vi "VI Tree.vi"   [LabVIEW 2010, in "Lake Shore 335.lvlib"]
doc: "This is the instrument driver for the Lake Shore Model 335 Temperature Controller. The VI Tree displays all the user-callable VIs of the instrument driver in an organized table."
uses:
  <instrlib>/Lake Shore 335/Lake Shore 335.lvlib
  <instrlib>/Lake Shore 335/Public/Data/Sensor Data (Single Reading).vi
panel:
  # "(c) 2011 Lake Shore Cryotronics Inc.  ALL RIGHTS RESERVED."
  # "SEE DIAGRAM\nFOR VI TREE."
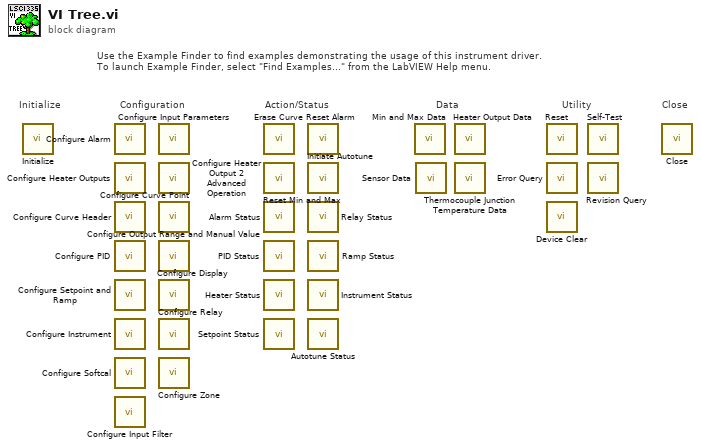
[diagram p0: block diagram]
diagram:
  # "Configuration"
  # "Utility"
  # "Data"
  # "Action/Status"
  # "Close"
  # "Initialize"
  # "Use the Example Finder to find examples demonstrating the usage of this instrument driver.\nTo launch Example Finder, select \"Find Examples...\" from the LabVIEW Help menu."
  n1 = call <instrlib>:"Initialize.vi"() -> ()  [unwired: 10 in, 2 out]
  n2 = call <instrlib>:"Configure Alarm.vi"() -> ()  [unwired: 14 in, 2 out]
  n3 = call <instrlib>:"Configure Heater Outputs.vi"() -> ()  [unwired: 18 in, 2 out]
  n4 = call <instrlib>:"Configure Curve Header.vi"() -> ()  [unwired: 14 in, 2 out]
  n5 = call <instrlib>:"Configure PID.vi"() -> ()  [unwired: 14 in, 2 out]
  n6 = call <instrlib>:"Configure Setpoint and Ramp.vi"() -> ()  [unwired: 14 in, 2 out]
  n7 = call <instrlib>:"Configure Instrument.vi"() -> ()  [unwired: 14 in, 2 out]
  n8 = call <instrlib>:"Configure Softcal.vi"() -> ()  [unwired: 14 in, 2 out]
  n9 = call <instrlib>:"Configure Input Filter.vi"() -> ()  [unwired: 14 in, 2 out]
  n10 = call <instrlib>:"Configure Input Parameters.vi"() -> ()  [unwired: 14 in, 2 out]
  n11 = call <instrlib>:"Configure Heater Output 2 Advanced Operation.vi"() -> ()  [unwired: 14 in, 2 out]
  n12 = call <instrlib>:"Configure Curve Point.vi"() -> ()  [unwired: 14 in, 2 out]
  n13 = call <instrlib>:"Configure Output Range and Manual Value.vi"() -> ()  [unwired: 14 in, 2 out]
  n14 = call <instrlib>:"Configure Display.vi"() -> ()  [unwired: 14 in, 2 out]
  n15 = call <instrlib>:"Configure Relay.vi"() -> ()  [unwired: 14 in, 2 out]
  n16 = call <instrlib>:"Configure Zone.vi"() -> ()  [unwired: 18 in, 2 out]
  n17 = call <instrlib>:"Erase Curve.vi"() -> ()  [unwired: 10 in, 2 out]
  n18 = call <instrlib>:"Reset Min and Max.vi"() -> ()  [unwired: 10 in, 2 out]
  n19 = call <instrlib>:"Alarm Status.vi"() -> ()  [unwired: 8 in, 4 out]
  n20 = call <instrlib>:"PID Status.vi"() -> ()  [unwired: 7 in, 5 out]
  n21 = call <instrlib>:"Heater Status.vi"() -> ()  [unwired: 7 in, 5 out]
  n22 = call <instrlib>:"Setpoint Status.vi"() -> ()  [unwired: 9 in, 3 out]
  n23 = call <instrlib>:"Reset Alarm.vi"() -> ()  [unwired: 10 in, 2 out]
  n24 = call <instrlib>:"Initiate Autotune.vi"() -> ()  [unwired: 14 in, 2 out]
  n25 = call <instrlib>:"Relay Status.vi"() -> ()  [unwired: 9 in, 3 out]
  n26 = call <instrlib>:"Ramp Status.vi"() -> ()  [unwired: 7 in, 5 out]
  n27 = call <instrlib>:"Instrument Status.vi"() -> ()  [unwired: 5 in, 7 out]
  n28 = call <instrlib>:"Autotune Status.vi"() -> ()  [unwired: 6 in, 6 out]
  n29 = call <instrlib>:"Min and Max Data.vi"() -> ()  [unwired: 8 in, 4 out]
  n30 = call-poly <instrlib>:"Sensor Data.vi"() -> ()  [unwired: 9 in, 3 out]
  n31 = call <instrlib>:"Heater Output Data.vi"() -> ()  [unwired: 9 in, 3 out]
  n32 = call <instrlib>:"Thermocouple Junction Temperature Data.vi"() -> ()  [unwired: 9 in, 3 out]
  n33 = call <instrlib>:"Reset.vi"() -> ()  [unwired: 10 in, 2 out]
  n34 = call <instrlib>:"Error Query.vi"() -> ()  [unwired: 9 in, 3 out]
  n35 = call <instrlib>:"Device Clear.vi"() -> ()  [unwired: 10 in, 2 out]
  n36 = call <instrlib>:"Self-Test.vi"() -> ()  [unwired: 8 in, 4 out]
  n37 = call <instrlib>:"Revision Query.vi"() -> ()  [unwired: 5 in, 7 out]
  n38 = call <instrlib>:"Close.vi"() -> ()  [unwired: 11 in, 1 out]
